vi "Get Message Sent Event.vi"(8 "error in":errorcluster, 11 "ICommunicate in":refnum<class "ICommunicate.lvclass">) -> (0 "error out":errorcluster, 2 "Msg Sent Event":refnum<user-event>, 3 "ICommunicate out":refnum<class "ICommunicate.lvclass">)   [LabVIEW 2024, in "ICommunicate.lvclass"]
uses:
  ICommunicate.lvclass
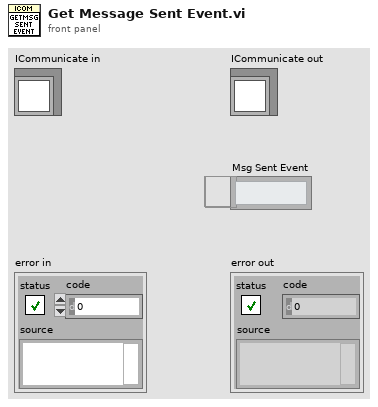
[diagram p1: front panel]
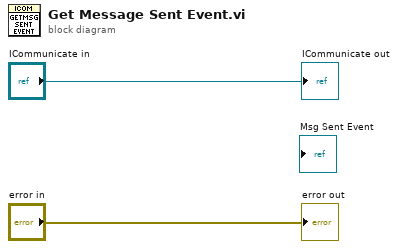
[diagram p0: block diagram]
diagram:
  "error out" <- "error in"
  "ICommunicate out" <- "ICommunicate in"
